vi "HRV_EEG.vi"() -> ()   [LabVIEW 2014]
uses:
  <vilib>/Utility/file.llb/Read From Spreadsheet File (I64).vi
  <vilib>/Utility/file.llb/Read From Spreadsheet File (DBL).vi
panel:
  in  "강제 Execution":bool
  out "HF":dbl[](graph)
  out "LF":dbl[](graph)
  out "VLF":dbl[](graph)
  in  "Mius_flash_order":path=path "C:/Users/Jaehong/Desktop/Classifiers/data/통합LDAs/kang/target_order.txt"
  in  "Order":path=path "C:/Users/Jaehong/Desktop/안전복지프로젝트/1차 2차 실험 데이터/Online_Data/강병훈_1_Training_Test/order.xls"
  in  "PPG_EEG":path=path "C:/Users/Jaehong/Desktop/안전복지프로젝트/1차 2차 실험 데이터/Online_Data/강병훈_1_Training_Test/강병훈PPGECG.xls"
  out "Executing":bool
  out "Target_icon":i64
  in  "Target_Total":path=path "C:/Users/Jaehong/Desktop/Classifiers/data/통합LDAs/kang/target_order.txt"
  in  "Icon_number":i32=1
  out "ERP_Graph":dbl[][](graph)
  in  "Trial_Number":i32=1
  in  "ERP_Total":path=path "C:/Users/Jaehong/Desktop/Classifiers/HRV_EEG/ERP_total/강병훈/ERP_total.txt"
  in  "stop":bool
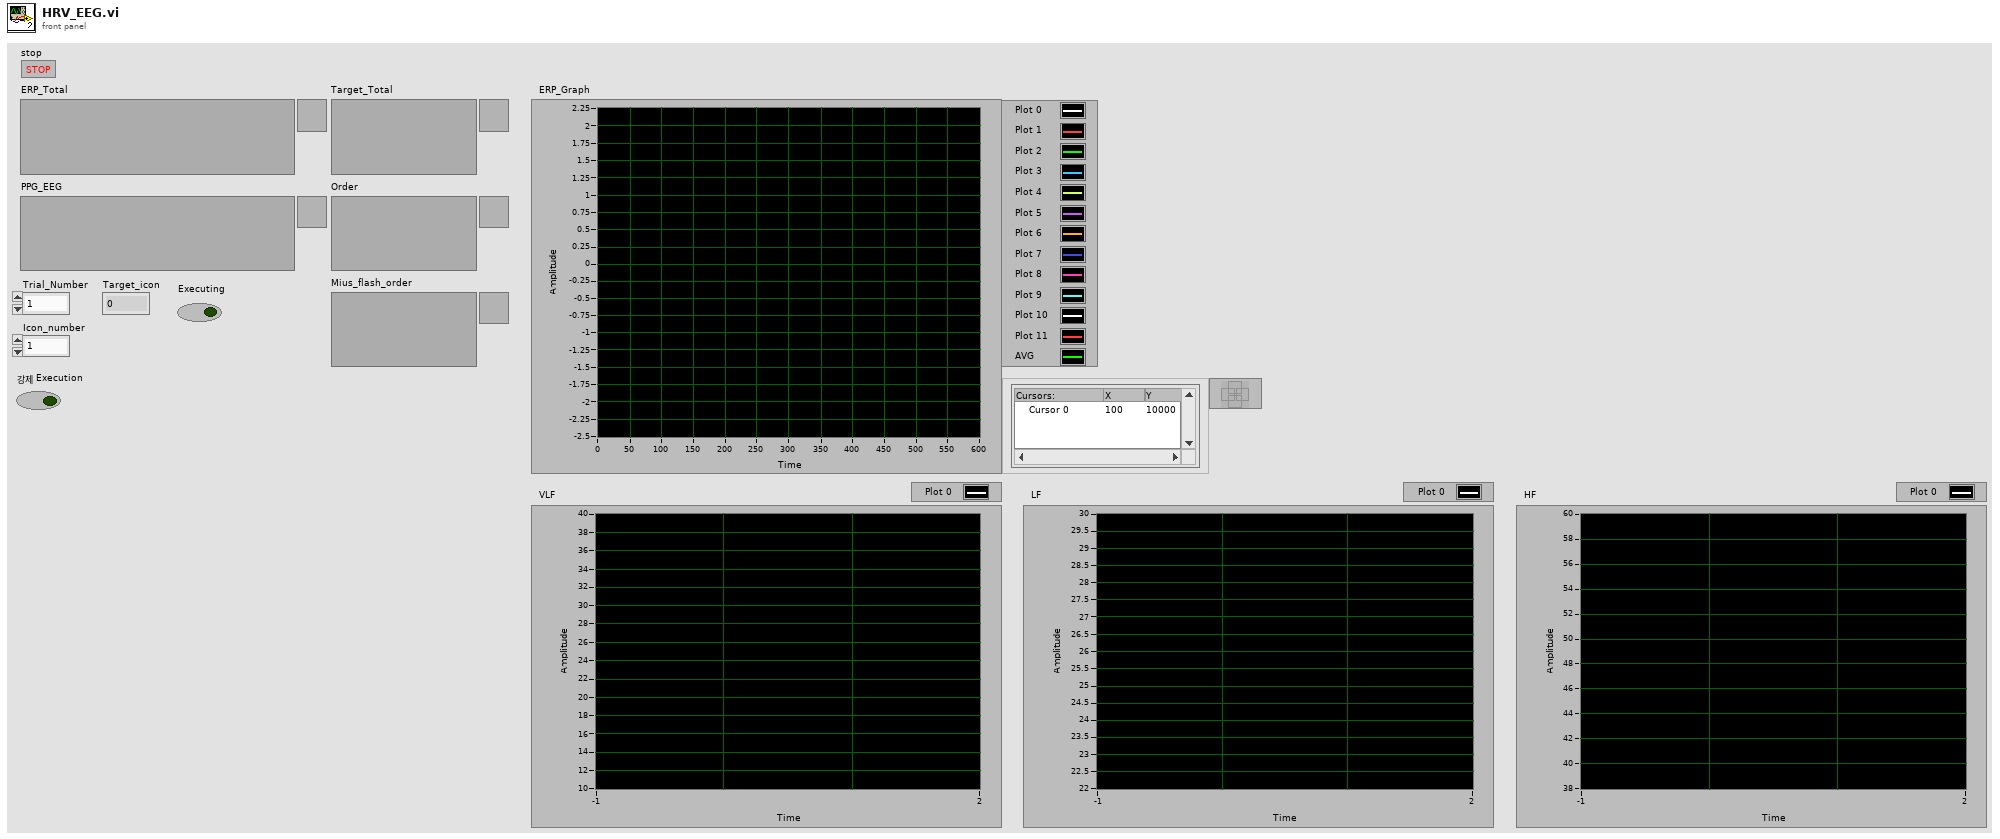
[diagram p1: front panel]
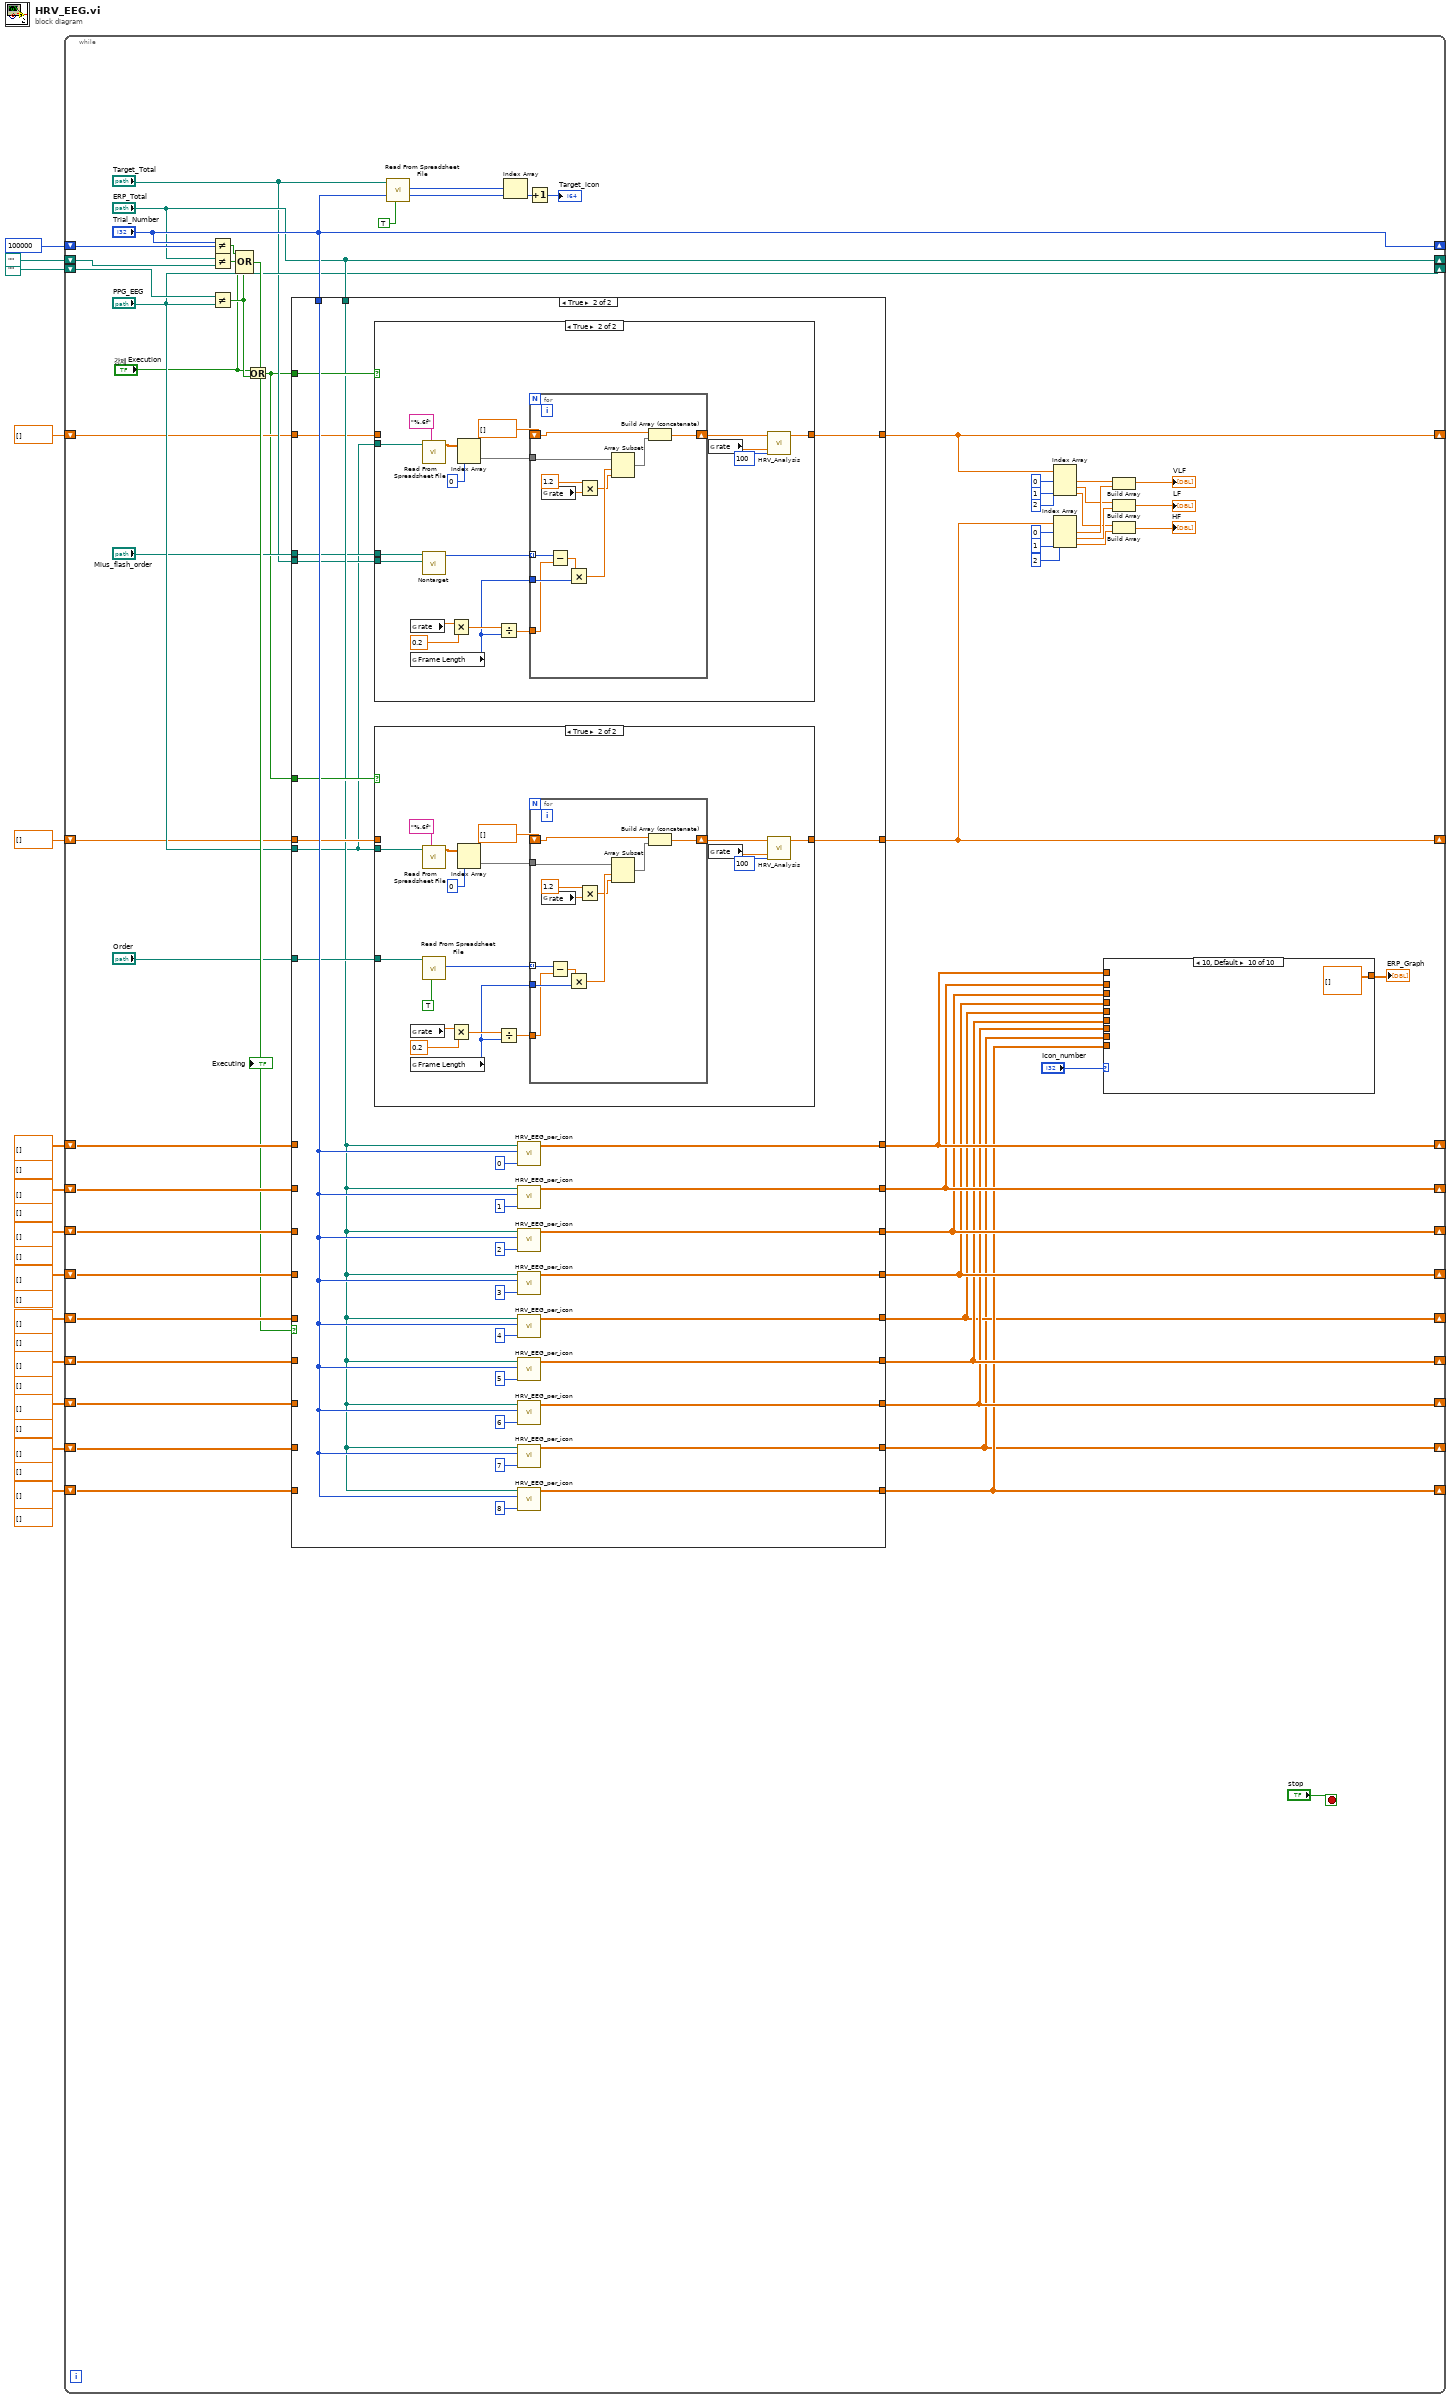
[diagram p0: block diagram]
diagram:
  (unwired) dbl[] [] ("PRV% (VLF, LF, HF)")
  (unwired) dbl[] [] ("PRV% (VLF, LF, HF)")
  (unwired) dbl[] [] ("PRV% (VLF, LF, HF)")
  (unwired) dbl[] [] ("PRV% (VLF, LF, HF)")
  (unwired) dbl[] [] ("PRV% (VLF, LF, HF)")
  (unwired) dbl[] [] ("PRV% (VLF, LF, HF)")
  (unwired) dbl[] [] ("PRV% (VLF, LF, HF)")
  (unwired) dbl[] [] ("PRV% (VLF, LF, HF)")
  (unwired) dbl[] [] ("PRV% (VLF, LF, HF)")
  n1 = while {
    shift-right: [w67] -> _
    shift-left: dbl[][] [] ("Icon1") -> [w60]
    shift-right: [w66] -> _
    shift-left: dbl[][] [] ("Icon1") -> [w59]
    shift-right: [w65] -> _
    shift-left: dbl[][] [] ("Icon1") -> [w58]
    shift-right: [w64] -> _
    shift-left: dbl[][] [] ("Icon1") -> [w57]
    shift-right: [w42] -> _
    shift-left: dbl[][] [] ("Icon1") -> [w56]
    shift-right: [w63] -> _
    shift-left: dbl[][] [] ("Icon1") -> [w55]
    shift-right: [w62] -> _
    shift-left: dbl[][] [] ("Icon1") -> [w54]
    shift-right: [w41] -> _
    shift-left: dbl[][] [] ("Icon1") -> [w53]
    shift-right: [w61] -> _
    shift-left: dbl[][] [] ("Icon1") -> [w52]
    shift-right: ["Trial_Number"] -> _
    shift-left: 100000 -> [w51]
    shift-right: ["ERP_Total"] -> _
    shift-left: path "" ("ERP_Total") -> [w48]
    shift-right: ["PPG_EEG"] -> _
    shift-left: path "" ("PPG_EEG") -> [w47]
    shift-right: [w34] -> _
    shift-left: dbl[] [] ("PRV% (VLF, LF, HF)") -> [w40]
    shift-right: [w35] -> _
    shift-left: dbl[] [] ("PRV% (VLF, LF, HF)") -> [w36]
    stop <- "stop" stop-if-true
    n2 = Not Equal?(x="Trial_Number", y=w51) -> (x != y?=w46:bool)
    n3 = Not Equal?(x="ERP_Total", y=w48) -> (x != y?=w39:bool)
    n4 = Not Equal?(x=w47, y="PPG_EEG") -> (x != y?=w18:bool)
    n5 = Compound Arithmetic op=OR(w46, w39, w18, "강제 Execution") -> (w45:bool)
    "Executing" <- w45
    n6 = Or(x="강제 Execution", y=w18) -> (x .or. y?=w16:bool)
    n7 = case shown="True" w45 {
      tunnel: "ERP_Total" -> [_ w90]
      tunnel: "Trial_Number" -> [_ w105]
      tunnel: [w84 w104] -> w67
      tunnel: [w83 w103] -> w66
      tunnel: [w82 w102] -> w65
      tunnel: [w81 w101] -> w64
      tunnel: [w80 w100] -> w42
      tunnel: [w79 w99] -> w63
      tunnel: [w78 w98] -> w62
      tunnel: [w77 w97] -> w41
      tunnel: [w76 w96] -> w61
      tunnel: w60 -> [w84 _]
      tunnel: w59 -> [w83 _]
      tunnel: w58 -> [w82 _]
      tunnel: w57 -> [w81 _]
      tunnel: w56 -> [w80 _]
      tunnel: w55 -> [w79 _]
      tunnel: w54 -> [w78 _]
      tunnel: w53 -> [w77 _]
      tunnel: w52 -> [w76 _]
      tunnel: "PPG_EEG" -> [_ w85]
      tunnel: "Order" -> [_ w95]
      tunnel: [w75 w94] -> w34
      tunnel: w40 -> [w75 w93]
      tunnel: w16 -> [_ w92]
      tunnel: w16 -> [_ w91]
      tunnel: "Mius_flash_order" -> [_ w89]
      tunnel: "Target_Total" -> [_ w88]
      tunnel: [w74 w87] -> w35
      tunnel: w36 -> [w74 w86]
      frame False {
      }
      frame True {
        n8 = case shown="True" w91 {
          tunnel: w85 -> [_ w130]
          tunnel: w89 -> [_ w129]
          tunnel: [w115 w117] -> w87
          tunnel: w86 -> [w115 _]
          tunnel: w88 -> [_ w116]
          frame False {
          }
          frame True {
            n9 = global read "Control_Panel.vi" "rate"() -> (w126:dbl)
            n10 = global read "Control_Panel.vi" "Frame Length"() -> (w124:i32)
            n11 = call-poly <vilib>:"Read From Spreadsheet File.vi"("format (%.3f)"="%.6f", "file path (dialog if empty)"=w130) -> ("all rows"=w132:dbl[][])  [unwired: 5 in, 4 out]
            n12 = call "Nontarget.vi"("Target_Total"=w116, "Mius_flash_order"=w129) -> ("Nontarget_order"=w128:i64[])  [unwired: 9 in]
            n13 = Multiply(x=w126, y=0.2) -> (x*y=w125:dbl)
            n14 = Index Array(array=w132, index (col)=0 ("index")) -> (element=w122:dbl[])  [unwired: 1 in]
            n15 = Divide(x=w125, y=w124) -> (x/y=w123:dbl)
            n16 = for {
              tunnel: w128 -> [w144] mode=indexing
              tunnel: w124 -> [w143]
              tunnel: w123 -> [w142]
              tunnel: w122 -> [w141]
              shift-right: [w135] -> w118
              shift-left: dbl[] [] -> [w134]
              n17 = global read "Control_Panel.vi" "rate"() -> (w139:dbl)
              n18 = Subtract(x=w144, y=w142) -> (x-y=w145:dbl)
              n19 = Multiply(x=w145, y=w143) -> (x*y=w140:dbl)
              n20 = Multiply(x=1.2, y=w139) -> (x*y=w137:dbl)
              n21 = Array Subset(array=w141, index=w140, length=w137) -> (w136:dbl[])
              n22 = Build Array (concatenate)(w134, w136) -> (w135:dbl[])
            }
            n23 = global read "Control_Panel.vi" "rate"() -> (w119:dbl)
            n24 = call "HRV_Analysis.vi"("Frame Length"=100, "Sample Rate"=w119, "PPG_Data"=w118) -> ("PRV% (VLF, LF, HF)"=w117:dbl[])  [unwired: 7 in, 1 out]
          }
        }
        n25 = case shown="True" w92 {
          tunnel: w85 -> [_ w161]
          tunnel: w95 -> [_ w159]
          tunnel: [w146 w147] -> w94
          tunnel: w93 -> [w146 _]
          frame False {
          }
          frame True {
            n26 = global read "Control_Panel.vi" "rate"() -> (w156:dbl)
            n27 = global read "Control_Panel.vi" "Frame Length"() -> (w154:i32)
            n28 = call-poly <vilib>:"Read From Spreadsheet File.vi"("format (%.3f)"="%.6f", "file path (dialog if empty)"=w161) -> ("all rows"=w163:dbl[][])  [unwired: 5 in, 4 out]
            n29 = call-poly <vilib>:"Read From Spreadsheet File.vi"("transpose (no:F)"=TRUE, "file path (dialog if empty)"=w159) -> ("first row"=w158:i64[])  [unwired: 5 in, 4 out]
            n30 = Multiply(x=w156, y=0.2) -> (x*y=w155:dbl)
            n31 = Index Array(array=w163, index (col)=0 ("index")) -> (element=w152:dbl[])  [unwired: 1 in]
            n32 = Divide(x=w155, y=w154) -> (x/y=w153:dbl)
            n33 = for {
              tunnel: w158 -> [w175] mode=indexing
              tunnel: w154 -> [w174]
              tunnel: w153 -> [w173]
              tunnel: w152 -> [w172]
              shift-right: [w166] -> w148
              shift-left: dbl[] [] -> [w165]
              n34 = global read "Control_Panel.vi" "rate"() -> (w170:dbl)
              n35 = Subtract(x=w175, y=w173) -> (x-y=w176:dbl)
              n36 = Multiply(x=w176, y=w174) -> (x*y=w171:dbl)
              n37 = Multiply(x=1.2, y=w170) -> (x*y=w168:dbl)
              n38 = Array Subset(array=w172, index=w171, length=w168) -> (w167:dbl[])
              n39 = Build Array (concatenate)(w165, w167) -> (w166:dbl[])
            }
            n40 = global read "Control_Panel.vi" "rate"() -> (w149:dbl)
            n41 = call "HRV_Analysis.vi"("Frame Length"=100, "Sample Rate"=w149, "PPG_Data"=w148) -> ("PRV% (VLF, LF, HF)"=w147:dbl[])  [unwired: 7 in, 1 out]
          }
        }
        n42 = call "HRV_EEG_per_icon.vi"("Icon Number"=0, "Trial_Number"=w105, "ERP_Total"=w90) -> ("Icon1"=w104:dbl[][])  [unwired: 8 in]
        n43 = call "HRV_EEG_per_icon.vi"("Icon Number"=1, "Trial_Number"=w105, "ERP_Total"=w90) -> ("Icon1"=w103:dbl[][])  [unwired: 8 in]
        n44 = call "HRV_EEG_per_icon.vi"("Icon Number"=2, "Trial_Number"=w105, "ERP_Total"=w90) -> ("Icon1"=w102:dbl[][])  [unwired: 8 in]
        n45 = call "HRV_EEG_per_icon.vi"("Icon Number"=3, "Trial_Number"=w105, "ERP_Total"=w90) -> ("Icon1"=w101:dbl[][])  [unwired: 8 in]
        n46 = call "HRV_EEG_per_icon.vi"("Icon Number"=4, "Trial_Number"=w105, "ERP_Total"=w90) -> ("Icon1"=w100:dbl[][])  [unwired: 8 in]
        n47 = call "HRV_EEG_per_icon.vi"("Icon Number"=5, "Trial_Number"=w105, "ERP_Total"=w90) -> ("Icon1"=w99:dbl[][])  [unwired: 8 in]
        n48 = call "HRV_EEG_per_icon.vi"("Icon Number"=6, "Trial_Number"=w105, "ERP_Total"=w90) -> ("Icon1"=w98:dbl[][])  [unwired: 8 in]
        n49 = call "HRV_EEG_per_icon.vi"("Icon Number"=7, "Trial_Number"=w105, "ERP_Total"=w90) -> ("Icon1"=w97:dbl[][])  [unwired: 8 in]
        n50 = call "HRV_EEG_per_icon.vi"("Icon Number"=8, "Trial_Number"=w105, "ERP_Total"=w90) -> ("Icon1"=w96:dbl[][])  [unwired: 8 in]
      }
    }
    n51 = call-poly <vilib>:"Read From Spreadsheet File.vi"("transpose (no:F)"=TRUE, "file path (dialog if empty)"="Target_Total") -> ("first row"=w69:i64[])  [unwired: 5 in, 4 out]
    n52 = Index Array(array=w69, index="Trial_Number") -> (element=w68:i64)
    n53 = Increment(x=w68) -> (x+1=→"Target_icon":i64)
    n54 = Index Array(array=w35, index #1=0 ("index"), index #2=1 ("index"), index #3=2 ("index")) -> (element #1=w27:dbl, element #2=w25:dbl, element #3=w22:dbl)
    n55 = Index Array(array=w34, index #1=0 ("index"), index #2=1 ("index"), index #3=2 ("index")) -> (element #1=w26:dbl, element #2=w24:dbl, element #3=w23:dbl)
    n56 = case shown="10, Default" "Icon_number" {
      tunnel: w67 -> [w177 _ _ _ _ _ _ _ _ _]
      tunnel: w66 -> [_ w178 _ _ _ _ _ _ _ _]
      tunnel: w65 -> [_ _ w179 _ _ _ _ _ _ _]
      tunnel: w64 -> [_ _ _ w180 _ _ _ _ _ _]
      tunnel: w42 -> [_ _ _ _ w181 _ _ _ _ _]
      tunnel: w63 -> [_ _ _ _ _ w182 _ _ _ _]
      tunnel: w62 -> [_ _ _ _ _ _ w183 _ _ _]
      tunnel: w41 -> [_ _ _ _ _ _ _ w184 _ _]
      tunnel: w61 -> [_ _ _ _ _ _ _ _ w185 _]
      tunnel: [w177 w178 w179 w180 w181 w182 w183 w184 w185 dbl[][] [] ("Icon1")] -> w71
      frame 1 {
      }
      frame 2 {
      }
      frame 3 {
      }
      frame 4 {
      }
      frame 5 {
      }
      frame 6 {
      }
      frame 7 {
      }
      frame 8 {
      }
      frame 9 {
      }
      frame 10, Default {
      }
    }
    "ERP_Graph" <- w71
    n57 = Build Array(w27, w26) -> (→"VLF":dbl[])
    n58 = Build Array(w25, w24) -> (→"LF":dbl[])
    n59 = Build Array(w22, w23) -> (→"HF":dbl[])
  }
